vi "Remove from Application MUXList.vi"(8 "error in (no error)":errorcluster, 10 "Source":string, 11 "SLSC Switch in":refnum<class "SLSC Switch.lvclass">) -> (0 "error out":errorcluster, 3 "SLSC Switch out":refnum<class "SLSC Switch.lvclass">)   [LabVIEW 2015, in "SLSC Switch.lvlib" / "SLSC Switch.lvclass"]
uses:
  SLSC Switch.lvclass
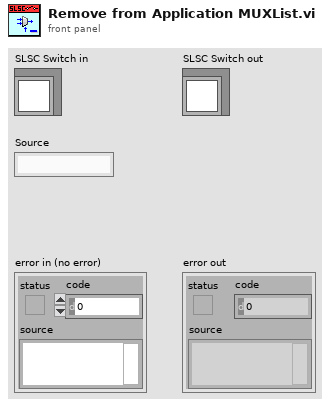
[diagram p1: front panel]
types:
  T1 = typedef "SLSC Switch.lvlib/SLSC Switch.lvclass/MuxList Entry.ctl" = cluster{"Source":string, "Destinations":string[]}
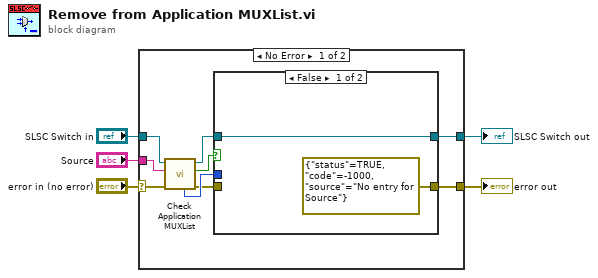
[diagram p0: block diagram]
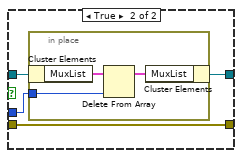
[diagram p2: hidden frame]
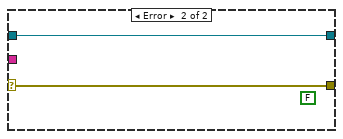
[diagram p3: hidden frame]
diagram:
  n1 = case shown="No Error" "error in (no error)" {
    selector: "error in (no error)" -> [w8 w25]
    tunnel: [w7 w25] -> w4
    tunnel: [w14 w24] -> w2
    tunnel: "SLSC Switch in" -> [w13 w24]
    tunnel: "Source" -> [w11 _]
    frame No Error {
      n2 = call "Check Application MUXList.vi"("error in (no error)"=w8, "Source"=w11, "SLSC Switch in"=w13) -> ("error out"=w6:errorcluster, "found?"=w9:bool, "SLSC Switch out"=w12:refnum<class "SLSC Switch.lvclass">, "index"=w10:i32)  [unwired: 4 in, 1 out]
      n3 = case shown="False" w9 {
        tunnel: [w16 w20] -> w14
        tunnel: w12 -> [w16 w19]
        tunnel: w10 -> [_ w18]
        tunnel: [errorcluster {"status"=TRUE, "code"=-1000, "source"="No entry for Source"} ("error out") w17] -> w7
        tunnel: w6 -> [_ w17]
        frame False {
        }
        frame True {
          n4 = in-place {
            in-place-border: w18 -> [w21]
            n5 = in-place-cluster #1(w19) -> ("MuxList"=w23:T1[])
            n6 = Delete From Array(array=w23, index=w21) -> (array with subset deleted=w22:T1[])  [unwired: 1 in, 1 out]
            n7 = in-place-cluster #1("MuxList"=w22) -> (w20:refnum<class "SLSC Switch.lvclass">)
          }
        }
      }
    }
    frame Error {
      (unwired) FALSE
    }
  }
  "error out" <- w4
  "SLSC Switch out" <- w2
